vi "Integral timescale scaling factor.vi"(1 "Integration threshold (0...1)":dbl min=0.0 max=1.0) -> (0 "Integral timescale scaling factor":dbl=1.0)   [LabVIEW 2016]
panel:
  # "Obtained via numerical simulation of gaussian random variable"
  # "PN 21/03/2017"
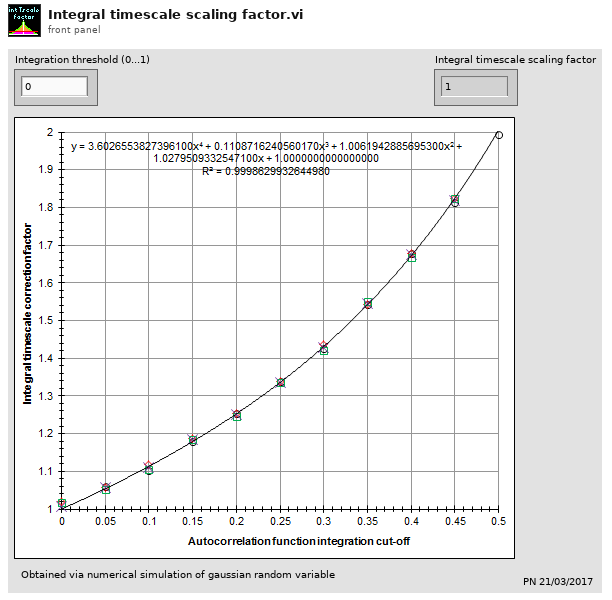
[diagram p1: front panel]
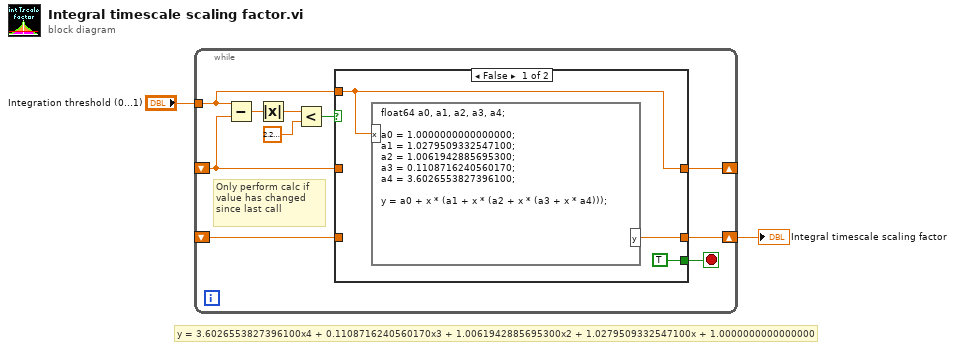
[diagram p0: block diagram]
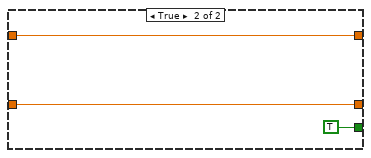
[diagram p2: hidden frame]
diagram:
  # "y = 3.6026553827396100x4 + 0.1108716240560170x3 + 1.0061942885695300x2 + 1.0279509332547100x + 1.0000000000000000"
  n1 = while {
    shift-right: [w4] -> _
    shift-left: _ -> [w5]
    tunnel: "Integration threshold (0...1)" -> [w6]
    shift-right: [w8] -> w1
    shift-left: _ -> [w7]
    stop <- w3 stop-if-true
    # "Only perform calc if value has changed since last call"
    n2 = Subtract(x=w6, y=w5) -> (x-y=w12:dbl)
    n3 = Absolute Value(x=w12) -> (abs(x)=w11:dbl)
    n4 = Less?(x=w11, y=2.220446049250313e-16) -> (x < y?=w9:bool)
    n5 = case shown="False" w9 {
      tunnel: [w15 w18] -> w8
      tunnel: w7 -> [_ w18]
      tunnel: w6 -> [w14 _]
      tunnel: [w14 w17] -> w4
      tunnel: w5 -> [_ w17]
      tunnel: [TRUE TRUE] -> w3
      frame False {
        n6 = formula code="float64 a0, a1, a2, a3, a4;\n\na0 = 1.0000000000000000;\na1 = 1.0279509332547100;\na2 = 1.0061942885695300;\na3 = 0.1108716240560170;\na4 = 3.6026553827396100;\n\ny = a0 + x * (a1 + x * (a2 + x * (a3 + x * a4)));"("x"=w14) -> ("y"=w15:dbl)
      }
      frame True {
      }
    }
  }
  "Integral timescale scaling factor" <- w1
